vi "correcaoCurva.vi"() -> ()   [LabVIEW 2012]
panel:
  in  "Temperatura desejada":dbl
  in  "Irradiância desejada":dbl
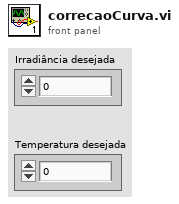
[diagram p1: front panel]
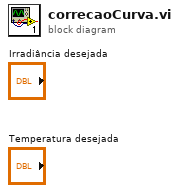
[diagram p0: block diagram]
diagram:
